vi "Launch.vi"(8 "error in (no error)":errorcluster, 10 "Mediator":refnum<class "IMediator.lvclass">, 11 "MediatorBusMonitor in":refnum<class "MediatorBusMonitor.lvclass">) -> (0 "error out":errorcluster, 1 "Bus Monitor Enqueuer":refnum<class "Message Enqueuer.lvclass">, 2 "Mediator Out":refnum<class "IMediator.lvclass">, 3 "Notification Msg Type":refnum<class "Notification Msg.lvclass">)   [LabVIEW 2017, in "Mediator.lvlib" / "MediatorBusMonitor.lvclass"]
uses:
  MediatorBusMonitor.lvclass
  C:/Program Files (x86)/National Instruments/LabVIEW 2017/vi.lib/ActorFramework/Actor/Actor.lvclass
  IMediator/IMediator/IMediator.lvclass
  <vilib>/ActorFramework/Message Enqueuer/Message Enqueuer.lvclass
  gpm_packages/@cs/transport/Source/Concrete/ActorMessageTransport/Notification Msg/Notification Msg.lvclass
  MediatorBusMonitor Messages/Bus Monitor Notification Msg/Bus Monitor Notification Msg.lvclass
  C:/Git/mva-framework/gpm_packages/@cs/transport/Source/Concrete/ActorMessageTransport/Notification Msg/Notification Msg.lvclass
  <vilib>/ActorFramework/Actor/Actor.lvclass
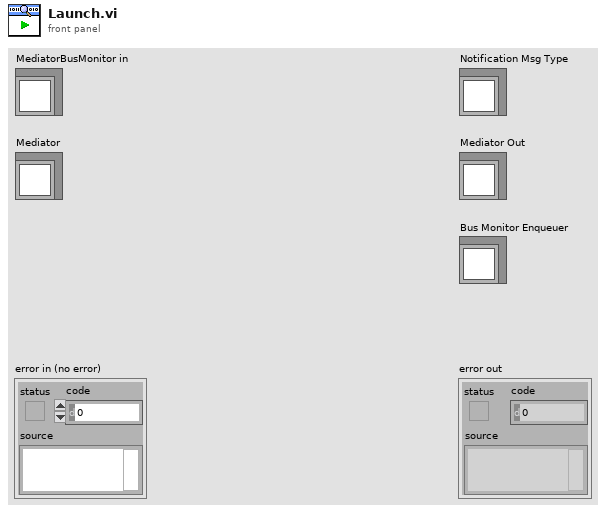
[diagram p1: front panel]
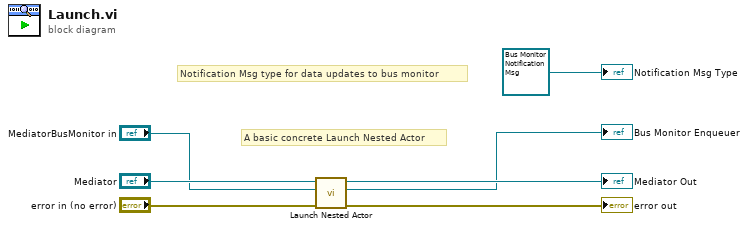
[diagram p0: block diagram]
diagram:
  # "Notification Msg type for data updates to bus monitor"
  # "A basic concrete Launch Nested Actor"
  n1 = call <vilib>:"Launch Nested Actor.vi"("error in (no error)"="error in (no error)", "Nested Actor"="MediatorBusMonitor in", "Caller Actor in"="Mediator") -> ("error out"=→"error out":errorcluster, "Nested Actor's Enqueuer"=→"Bus Monitor Enqueuer":refnum<class "Message Enqueuer.lvclass">, "Caller Actor out"=→"Mediator Out":refnum<class "IMediator.lvclass">)  [unwired: 6 in]
  "Notification Msg Type" <- refnum<class "Bus Monitor Notification Msg.lvclass"> refnum ("Mediator.lvlib:Bus Monitor Notification Msg.lvclass")
